vi "PosToLO.vi"(0 "Convertion":T1, 1 "a":dbl) -> (7 "P(a)":dbl)   [LabVIEW 2013]
uses:
  Convertion.ctl
  <vilib>/Analysis/polynomials.llb/Scalar Polynomial Evaluation (DBL).vi
  <vilib>/Analysis/NI_AALPro.lvlib
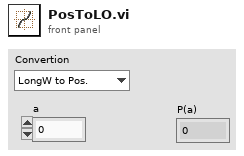
[diagram p1: front panel]
types:
  T1 = typedef "Convertion.ctl" = enum16{"LongW to Pos.", "Pos. To longW"}
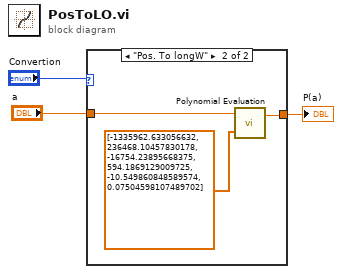
[diagram p0: block diagram]
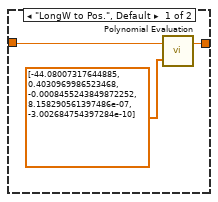
[diagram p2: hidden frame]
diagram:
  n1 = case shown="\"Pos. To longW\"" "Convertion" {
    tunnel: "a" -> [w5 w8]
    tunnel: [w4 w7] -> w1
    frame "LongW to Pos.", Default {
      n2 = call-poly <vilib>:"Polynomial Evaluation.vi"("P(x)"=dbl[] [-44.08007317644885, 0.4030969986523468, -0.0008455243849872252, 8.158290561397486e-07, -3.002684754397284e-10] ("Polynomial Coefficients"), "a"=w5) -> ("P(a)"=w4:dbl)  [unwired: 1 out]
    }
    frame "Pos. To longW" {
      n3 = call-poly <vilib>:"Polynomial Evaluation.vi"("P(x)"=dbl[] [-1335962.633056632, 236468.10457830178, -16754.23895668375, 594.1869129009725, -10.549860848589574, 0.07504598107489702] ("Polynomial Coefficients"), "a"=w8) -> ("P(a)"=w7:dbl)  [unwired: 1 out]
    }
  }
  "P(a)" <- w1
